vi "AnalysisData.vi"() -> ()   [LabVIEW 2011]
panel:
  out "RunState":string
  out "PowerState":string
  in  "数组":string[][](array[string])
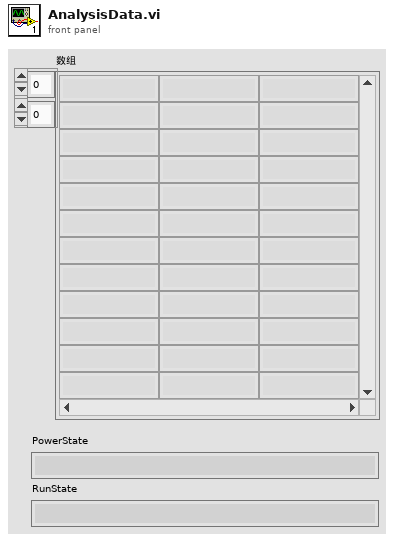
[diagram p1: front panel]
types:
  T1 = enum16{"RINSE_INIT", "RINSE_DRAIN", "RINSE_SUDS_REDUCTION", "RINSE_SPIN", "RINSE_WATERSUPPLY", "RINSE_RINSE", "RINSE_REMOVE_SUDS", "RINSE_END"}
  T2 = enum16{"WASH_INIT", "WASH_DRUMWASHWATER", "WASH_DRUMWASHRINSE", "WASH_DRUMWASHDRAIN", "WASH_WEIGHT", "WASH_DRUMWASHWEIGHT", "WASH_WATERSUPPLY", "WASH_WASH1", "WASH_WASH2", "WASH_WASH3", "WASH_WASH4", "WASH_WASH5", "WASH_WASH6", "WASH_MAGICSTEAM_DRAIN", "WASH_MAGICSTEAM_SUPPLY", "WASH_MAGICSTEAM_TUMBLE", "WASH_END"}
  T3 = enum16{"PREWASH_INIT", "PREWASH_WEIGHT", "PREWASH_WATERSUPPLY", "PREWASH_WASH1", "PREWASH_WASH2", "PREWASH_DRAIN", "PREWASH_SPIN", "PREWASH_END", "PREWASH_STEP_MAX"}
  T4 = enum16{"RESERVE_INIT", "RESERVE_WEIGHT", "RESERVE_RESERVE", "RESERVE_FIRST_DRAIN"}
  T5 = enum16{"INITPROGRESS_INIT", "INITPROGRESS_FIRST_DRAIN_INIT", "INITPROGRESS_FIRST_DRAIN_ACTION"}
  T6 = enum16{"PROGRESS_INITIAL", "PROGRESS_RESERVE", "PROGRESS_PREWASH", "PROGRESS_WASH", "PROGRESS_RINSE", "PROGRESS_FINALSPIN", "PROGRESS_DRY", "PROGRESS_AIRWASH", "PROGRESS_FINISH", "PROGRESS_END", "PROGRESS_MAX"}
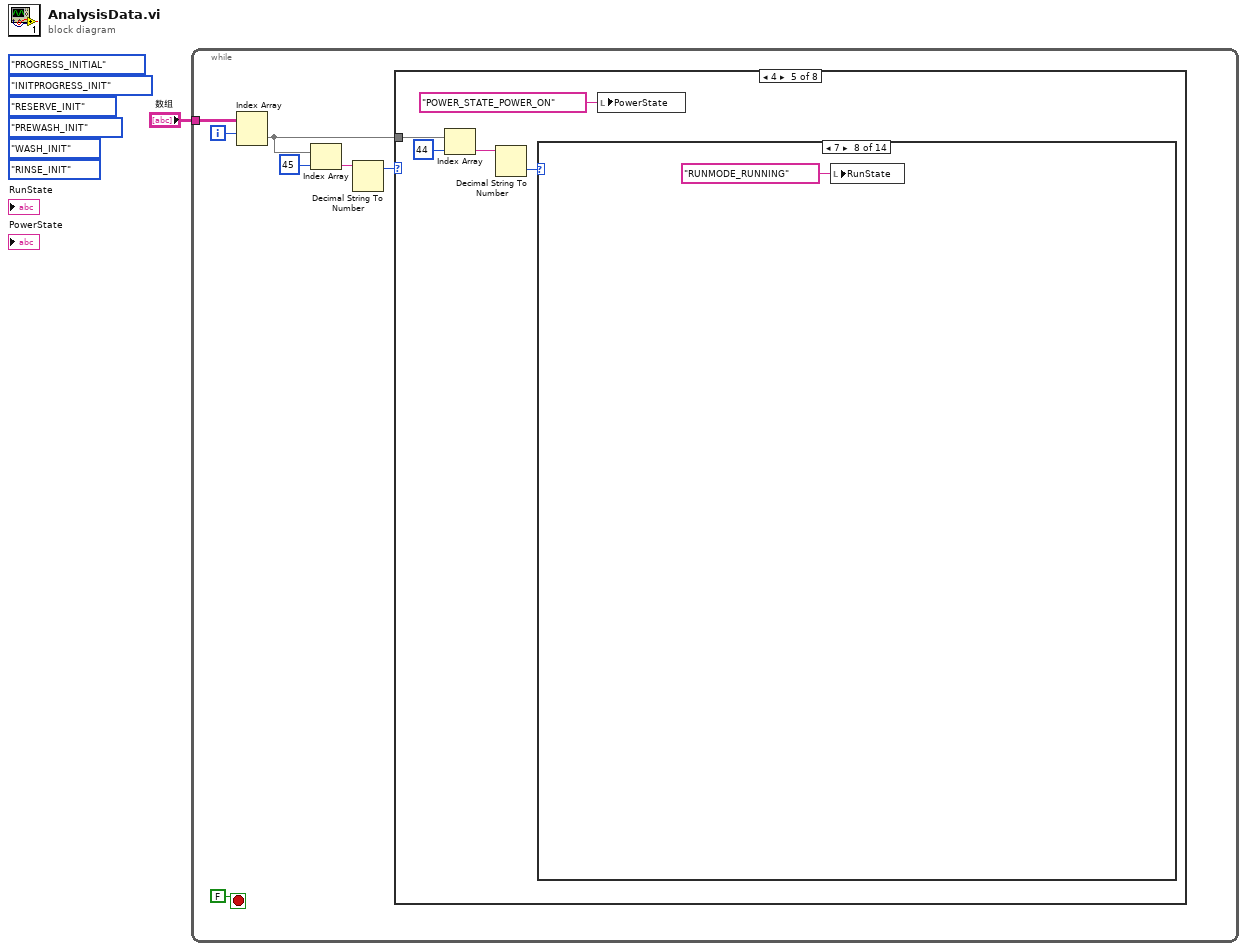
[diagram p0: block diagram]
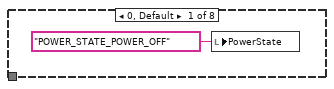
[diagram p2: hidden frame]
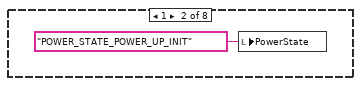
[diagram p3: hidden frame]
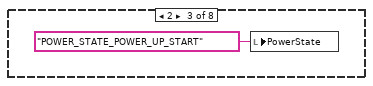
[diagram p4: hidden frame]
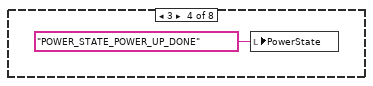
[diagram p5: hidden frame]
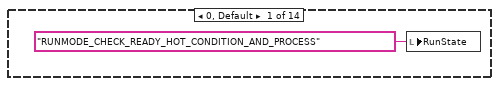
[diagram p6: hidden frame]
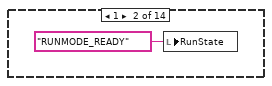
[diagram p7: hidden frame]
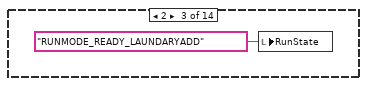
[diagram p8: hidden frame]
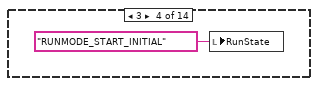
[diagram p9: hidden frame]
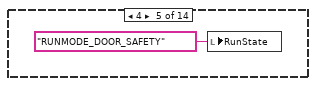
[diagram p10: hidden frame]
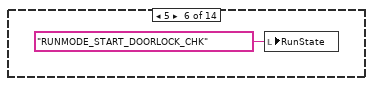
[diagram p11: hidden frame]
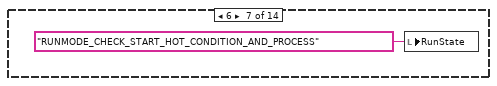
[diagram p12: hidden frame]
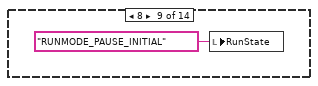
[diagram p13: hidden frame]
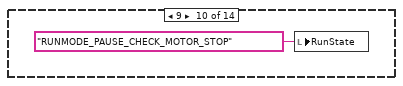
[diagram p14: hidden frame]
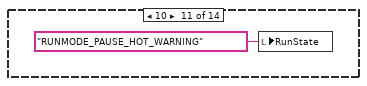
[diagram p15: hidden frame]
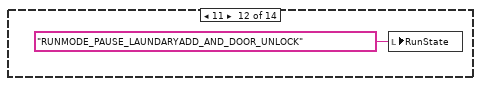
[diagram p16: hidden frame]
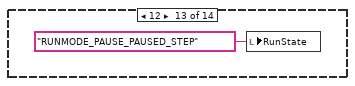
[diagram p17: hidden frame]
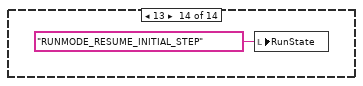
[diagram p18: hidden frame]
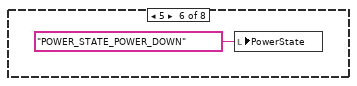
[diagram p19: hidden frame]
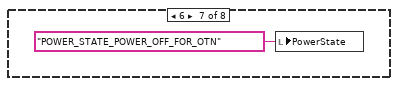
[diagram p20: hidden frame]
diagram:
  (unwired) T1."RINSE_INIT"
  (unwired) T2."WASH_INIT"
  (unwired) T3."PREWASH_INIT"
  (unwired) T4."RESERVE_INIT"
  (unwired) T5."INITPROGRESS_INIT"
  (unwired) T6."PROGRESS_INITIAL"
  n1 = while {
    tunnel: "数组" -> [w8]
    i -> [w7]
    stop <- FALSE stop-if-true
    n2 = Index Array(array=w8, index (row)=w7) -> (element=w3:string[])  [unwired: 1 in]
    n3 = Index Array(array=w3, index=45 ("索引")) -> (element=w5:string)
    n4 = Decimal String To Number(string=w5) -> (offset past number=w4:i32)  [unwired: 2 in, 1 out]
    n5 = case shown="4" w4 {
      tunnel: w3 -> [_ _ _ _ w16 _ _ _]
      frame 0, Default {
        n6 = local write "PowerState"("POWER_STATE_POWER_OFF" ("PowerState")) -> ()
      }
      frame 1 {
        n7 = local write "PowerState"("POWER_STATE_POWER_UP_INIT" ("PowerState")) -> ()
      }
      frame 2 {
        n8 = local write "PowerState"("POWER_STATE_POWER_UP_START" ("PowerState")) -> ()
      }
      frame 3 {
        n9 = local write "PowerState"("POWER_STATE_POWER_UP_DONE" ("PowerState")) -> ()
      }
      frame 4 {
        n10 = Index Array(array=w16, index=44 ("索引")) -> (element=w14:string)
        n11 = Decimal String To Number(string=w14) -> (number=w13:i32)  [unwired: 2 in, 1 out]
        n12 = case shown="7" w13 {
          frame 0, Default {
            n13 = local write "RunState"("RUNMODE_CHECK_READY_HOT_CONDITION_AND_PROCESS" ("RunState")) -> ()
          }
          frame 1 {
            n14 = local write "RunState"("RUNMODE_READY" ("RunState")) -> ()
          }
          frame 2 {
            n15 = local write "RunState"("RUNMODE_READY_LAUNDARYADD" ("RunState")) -> ()
          }
          frame 3 {
            n16 = local write "RunState"("RUNMODE_START_INITIAL" ("RunState")) -> ()
          }
          frame 4 {
            n17 = local write "RunState"("RUNMODE_DOOR_SAFETY" ("RunState")) -> ()
          }
          frame 5 {
            n18 = local write "RunState"("RUNMODE_START_DOORLOCK_CHK" ("RunState")) -> ()
          }
          frame 6 {
            n19 = local write "RunState"("RUNMODE_CHECK_START_HOT_CONDITION_AND_PROCESS" ("RunState")) -> ()
          }
          frame 7 {
            n20 = local write "RunState"("RUNMODE_RUNNING" ("RunState")) -> ()
          }
          frame 8 {
            n21 = local write "RunState"("RUNMODE_PAUSE_INITIAL" ("RunState")) -> ()
          }
          frame 9 {
            n22 = local write "RunState"("RUNMODE_PAUSE_CHECK_MOTOR_STOP" ("RunState")) -> ()
          }
          frame 10 {
            n23 = local write "RunState"("RUNMODE_PAUSE_HOT_WARNING" ("RunState")) -> ()
          }
          frame 11 {
            n24 = local write "RunState"("RUNMODE_PAUSE_LAUNDARYADD_AND_DOOR_UNLOCK" ("RunState")) -> ()
          }
          frame 12 {
            n25 = local write "RunState"("RUNMODE_PAUSE_PAUSED_STEP" ("RunState")) -> ()
          }
          frame 13 {
            n26 = local write "RunState"("RUNMODE_RESUME_INITIAL_STEP" ("RunState")) -> ()
          }
        }
        n27 = local write "PowerState"("POWER_STATE_POWER_ON" ("PowerState")) -> ()
      }
      frame 5 {
        n28 = local write "PowerState"("POWER_STATE_POWER_DOWN" ("PowerState")) -> ()
      }
      frame 6 {
        n29 = local write "PowerState"("POWER_STATE_POWER_OFF_FOR_OTN" ("PowerState")) -> ()
      }
      frame 7 {
        n30 = local write "PowerState"("POWER_STATE_POWER_SLEEP_MODE" ("PowerState")) -> ()
      }
    }
  }
